vi "Route Switch.vi"(8 "error in":errorcluster, 9 "Route to:":T1=enum."Channel 2", 10 "Route From:":T1, 11 "LTB-1 in":refnum<class "LTB-1.lvclass">) -> (0 "error out":errorcluster, 3 "LTB-1 out":refnum<class "LTB-1.lvclass">)   [LabVIEW 2018]
doc: "This is a dynamically dispatched VI. The child class will set the optical signal path through the switch. EXFO switches can handle up to 16 channels. Be sure to verify if there are less than 16 channels that the input values are within the range of installed switch routes.\n\nAuthor: Ron Dexter\nCompany: Luminar\nModified: 5/20/2018"
uses:
  PPLs/EXFO/Parent/EXFO.lvlibp/Private/Switch Channels.ctl
  PPLs/EXFO/Parent/EXFO.lvlibp
  LTB-1.lvclass
  C:/AME Test Engineering/LabVIEW/PPLs/EXFO/Parent/EXFO.lvlibp/EXFO.lvclass
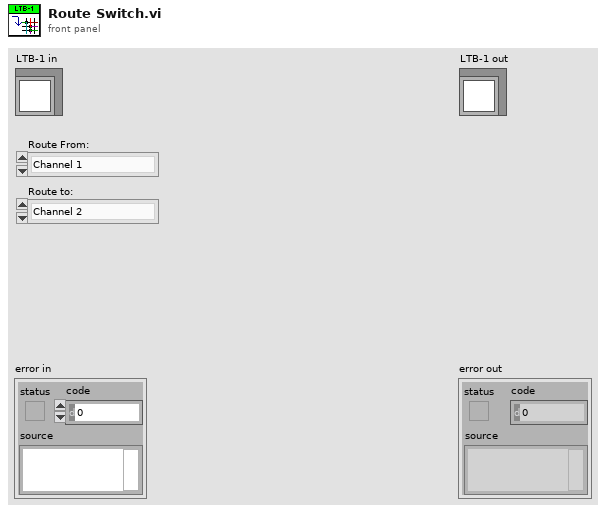
[diagram p1: front panel]
types:
  T1 = typedef "EXFO.lvlibp/Switch Channels.ctl" = enum16{"Channel 1", "Channel 2", "Channel 3", "Channel 4", "Channel 5", "Channel 6", "Channel 7", "Channel 8", "Channel 9", "Channel 10", "Channel 11", "Channel 12", "Channel 13", "Channel 14", "Channel 15", "Channel 16"}
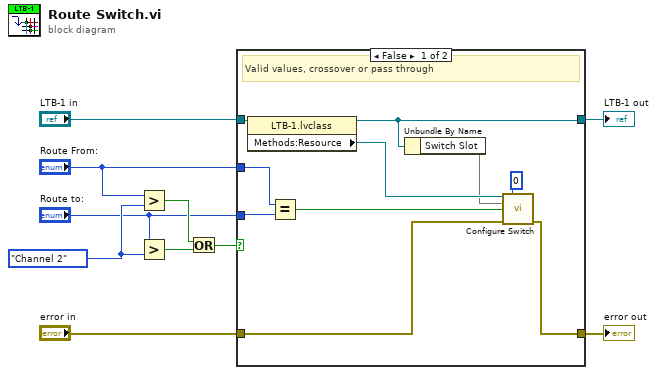
[diagram p0: block diagram]
diagram:
  w10 = Switch_Channels."Channel 2" ("y")
  n1 = Greater?(x="Route From:", y=w10) -> (0:w8:bool)
  n2 = Greater?(x="Route to:", y=w10) -> (0:w9:bool)
  n3 = Or(x=w8, y=w9) -> (x .or. y?=w7:bool)
  n4 = case shown="False" w7 {
    tunnel: [w15 w22] -> w6
    tunnel: "LTB-1 in" -> [w17 w22]
    tunnel: "error in" -> [w12 w21]
    tunnel: [w11 w21] -> w3
    tunnel: "Route to:" -> [w20 _]
    tunnel: "Route From:" -> [w19 _]
    frame False {
      # "Valid values, crossover or pass through"
      n5 = property class="LTB-1.lvclass"(reference=w17) -> (reference out=w15:refnum<class "LTB-1.lvclass">, "Methods:Resource"=w16:refnum<visa-resource-name>)  [unwired: 1 in, 1 out]
      n6 = Equal?(x=w19, y=w20) -> (x = y?=w18:bool)
      n7 = Unbundle By Name(w15) -> ("Switch Slot"=w14)
      n8 = call <instrlib>:"Configure Switch.vi"("VISA resource name"=w16, "Platform"=i16 0, "Module Slot Number (10)"=w14, "Enable Shutter State (F:OFF)"=w18, "error in (no error)"=w12) -> ("error out"=w11:errorcluster)  [unwired: 9 in, 1 out]
    }
    frame True {
      # "Invalid route option"
    }
  }
  "error out" <- w3
  "LTB-1 out" <- w6
